vi "Pigeon Yaw.vi"(8 "error in (no error)":errorcluster, 11 "Turret in":refnum<class "Turret.lvclass">) -> (0 "error out":errorcluster, 1 "Yaw":dbl, 3 "Turret out":refnum<class "Turret.lvclass">)   [LabVIEW 2019, in "Turret.lvlib" / "Turret.lvclass"]
uses:
  Turret.lvclass
  Turret.lvclass/Turret.ctl
  <vilib>/Rock Robotics/WPI/ThirdParty/Phoenix-LabVIEW/Pigeon IMU/CTRE_PigeonIMU_GetYPR.vi
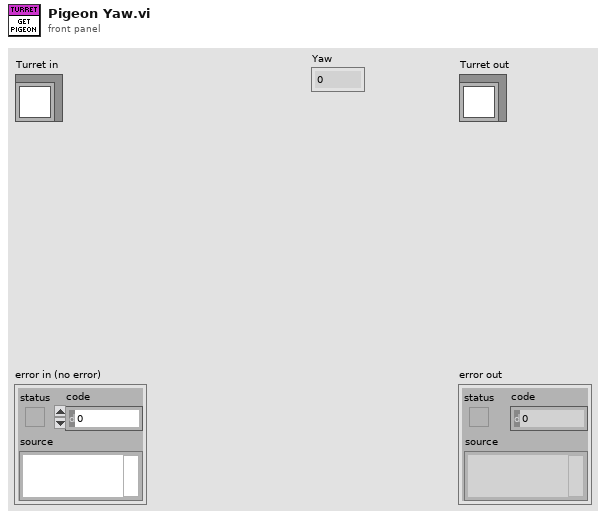
[diagram p1: front panel]
types:
  T1 = typedef "CTRE_PigeonIMU_DeviceRef.ctl" = cluster{"DeviceStatus":errorcluster, "Device Number":u8, "Type":T2, "Device ID":u32, "Handle":u64, "UsageFrame":u32, "Library Path":path}
  T2 = typedef "CTRE_PigeonIMU_ConnectionType.ctl" = u32
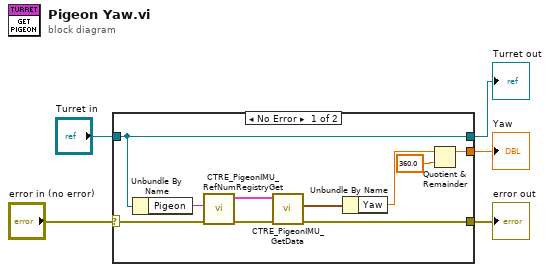
[diagram p0: block diagram]
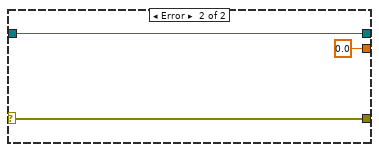
[diagram p2: hidden frame]
diagram:
  n1 = case shown="No Error" "error in (no error)" {
    selector: "error in (no error)" -> [w12 w18]
    tunnel: [w11 w18] -> w4
    tunnel: [w15 w17] -> w2
    tunnel: "Turret in" -> [w15 w17]
    tunnel: [w7 0.0] -> w1
    frame No Error {
      n2 = Unbundle By Name(w15) -> ("Pigeon"=w9:string)
      n3 = call <vilib>:"CTRE_PigeonIMU_RefNumRegistryGet.vi"("error in (no error)"=w12, "refnum name"=w9) -> ("error out"=w13:errorcluster, "PigeonIMUDevRef"=w14:T1)  [unwired: 8 in]
      n4 = call-poly <vilib>:"CTRE_PigeonIMU_GetData.vi"("error in (no error)"=w13, "PigeonIMUDevRef"=w14) -> ("error out"=w11:errorcluster, "Yaw Pitch Roll"=w10:cluster{"Yaw":dbl, "Pitch":dbl, "Roll":dbl})  [unwired: 7 in, 1 out]
      n5 = Unbundle By Name(w10) -> ("Yaw"=w8:dbl)
      n6 = Quotient & Remainder(x=w8, y=360.0) -> (x-y*floor(x/y)=w7:dbl)  [unwired: 1 out]
    }
    frame Error {
    }
  }
  "error out" <- w4
  "Turret out" <- w2
  "Yaw" <- w1
